vi "Pfeiffer-RVC300.ProcPeriodic.vi"(0 "i ref in":refnum<vi>, 3 "ms timeout (10000)":i32=10000, 5 "error in (no error)":errorcluster) -> (14 "i ref out":refnum<vi>, 17 "timed out":bool, 19 "error out":errorcluster)   [LabVIEW 2014, in "Pfeiffer-RVC300.lvlib"]
doc: "This method serves to periodically do things like reading values from the HW. Methods that should be executed periodically should be called from THIS methode. Add code here."
uses:
  Pfeiffer-RVC300.lvlib
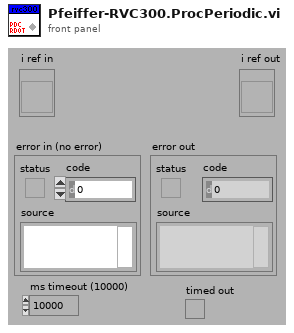
[diagram p1: front panel]
types:
  T1 = typedef "Pfeiffer-RVC300.lvlib/Pfeiffer-RVC300.i attribute.ctl" = cluster{"interfaceInitialized":bool, "VISAResource":refnum<visa-resource-name>, "WaitingTime":u32, "nomValues":T2, "actValues":T2}
  T2 = typedef "Pfeiffer-RVC300.lvlib/Pfeiffer-RVC300.parameters.ctl" = cluster{"regulationMode":T3, "valveType":string, "sensorType":string, "valveState":string, "flow":dbl, "pressure":dbl, "serviceIDs":cluster{"regulationModeID":i32, "valveTypeID":i32, "sensorTypeID":i32, "valveStateID":i32, "flowID":i32, "pressureID":i32}}
  T3 = typedef "Pfeiffer-RVC300.lvlib/Pfeiffer-RVC300.regulation mode.ctl" = enum16{"unknown", "Pressure", "Flow", "Wait"}
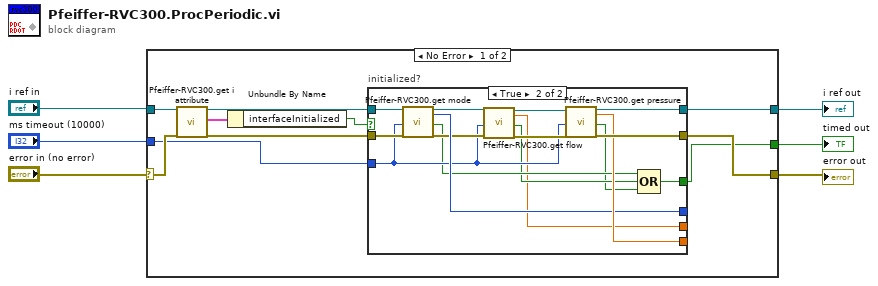
[diagram p0: block diagram]
diagram:
  n1 = case shown="No Error" "error in (no error)" {
    selector: "error in (no error)" -> [w16 w35]
    tunnel: "i ref in" -> [w15 w36]
    tunnel: "ms timeout (10000)" -> [w11 _]
    tunnel: [w9 w35] -> w3
    tunnel: [w8 _] -> w2
    tunnel: [w7 w36] -> w1
    frame No Error {
      n2 = call "Pfeiffer-RVC300.get i attribute.vi"("i ref in"=w15, "error in (no error)"=w16) -> ("i ref out"=w10:refnum<vi>, "i attribute"=w14:T1, "error out"=w12:errorcluster)  [unwired: 15 in]
      n3 = Unbundle By Name(w14) -> ("interfaceInitialized"=w13:bool)
      n4 = case "initialized?" shown="True" w13 {
        tunnel: w12 -> [w17 w34]
        tunnel: w11 -> [_ w23]
        tunnel: w10 -> [w18 w33]
        tunnel: [w17 w31] -> w9
        tunnel: [_ w30] -> w8
        tunnel: [w18 w32] -> w7
        tunnel: [_ w29] -> _
        tunnel: [_ w28] -> _
        tunnel: [_ w19] -> _
        frame False {
        }
        frame True {
          n5 = call "Pfeiffer-RVC300.get mode.vi"("i ref in"=w33, "ms timeout (10000)"=w23, "error in (no error)"=w34) -> ("i ref out"=w26:refnum<vi>, "regulationMode"=w28:T3, "timed out"=w22:bool, "error out"=w25:errorcluster)  [unwired: 13 in]
          n6 = call "Pfeiffer-RVC300.get flow.vi"("i ref in"=w26, "ms timeout (10000)"=w23, "error in (no error)"=w25) -> ("i ref out"=w27:refnum<vi>, "flow"=w19:dbl, "timed out"=w21:bool, "error out"=w24:errorcluster)  [unwired: 13 in]
          n7 = call "Pfeiffer-RVC300.get pressure.vi"("i ref in"=w27, "ms timeout (10000)"=w23, "error in (no error)"=w24) -> ("i ref out"=w32:refnum<vi>, "pressure"=w29:dbl, "timed out"=w20:bool, "error out"=w31:errorcluster)  [unwired: 13 in]
          n8 = Compound Arithmetic op=OR(w22, w21, w20) -> (w30:bool)
        }
      }
    }
    frame Error {
    }
  }
  "error out" <- w3
  "i ref out" <- w1
  "timed out" <- w2
